vi "init.vi"(8 "error in (no error)":errorcluster, 11 "Stepper in":refnum<class "Stepper.lvclass">) -> (0 "error out":errorcluster, 3 "Stepper out":refnum<class "Stepper.lvclass">)   [LabVIEW 2025, in "Stepper.lvclass"]
uses:
  Stepper.lvclass
  Stepper.lvclass/Stepper.ctl
  <vilib>/NI/Modbus Library/API/Wrapper/Create Serial Master.vi
  <vilib>/NI/Modbus Library/API/Wrapper/API Main.lvlib
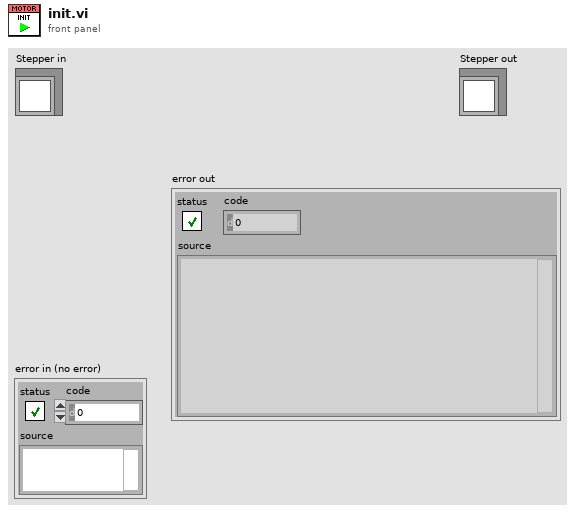
[diagram p1: front panel]
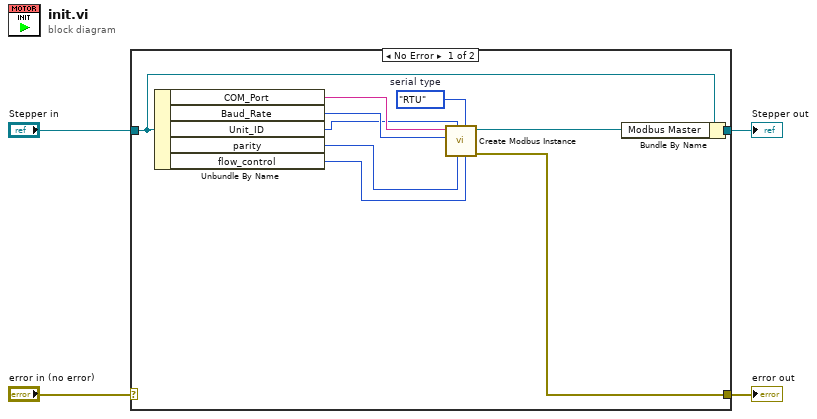
[diagram p0: block diagram]
diagram:
  n1 = case shown="No Error" "error in (no error)" {
    selector: "error in (no error)" -> [_ w16]
    tunnel: [w5 w16] -> w3
    tunnel: [w14 w15] -> w1
    tunnel: "Stepper in" -> [w13 w15]
    frame No Error {
      w9 = enum16{"RTU", "ASCII"}."RTU"  # serial type
      n2 = Unbundle By Name(w13) -> ("COM_Port"=w12:string, "Baud_Rate"=w11:u32, "Unit_ID"=w10:u8, "parity"=w8:u16, "flow_control"=w7:u16)
      n3 = call-poly <vilib>:"Create Modbus Instance.vi"("flow control (none)"=w7, "serial type"=w9, "parity (even)"=w8, "unit ID"=w10, "baud rate"=w11, "VISA resource name"=w12) -> ("error out"=w5:errorcluster, "serial master instance"=w6:refnum<class "Modbus Master.lvclass">)  [unwired: 4 in]
      n4 = Bundle By Name(cluster=w13, "Modbus Master"=w6) -> (w14:refnum<class "Stepper.lvclass">)
    }
    frame Error {
    }
  }
  "error out" <- w3
  "Stepper out" <- w1
